vi "Finish.vi"   [LabVIEW 2014]
doc: "This VI is called just before exiting. It is expected to close I/O refnum, save collected data, etc."
uses:
  <vilib>/Rock Robotics/WPI/Joystick/WPI_JoystickGetSetRefNum.vi
  <vilib>/Rock Robotics/WPI/RobotDrive/WPI_RobotDriveGetSetRefNum.vi
types:
  T1 = typedef "WPI_JoystickDevRef.ctl" = cluster{"Device":T2}
  T2 = typedef "WPI_JoystickDeviceEnum.ctl" = enum16{"USB 0", "USB 1", "USB 2", "USB 3", "USB 4", "USB 5"}
  T3 = typedef "WPI_RobotDriveDevRef.ctl" = cluster{"DevStatus":errorcluster, "Motors[]":T4[], "Square Inputs":bool, "Max Output":dbl}
  T4 = typedef "WPI_MotorControlDeviceRef.ctl" = cluster{"DeviceStatus":errorcluster, "Type":T5, "PWM":cluster{"Controller":T6, "PWM Channel":T7, "DeadBand":T8}, "CAN":cluster{"Device Number":u8, "Control Mode":T9, "Semaphore":T10, "Max Vout":dbl, "TalonSRX Control Mode":T11}, "Invert":bool, "TransformRef":T12, "InvTransformRef":T12}
  T5 = typedef "WPI_MotorControlType.ctl" = enum16{"PWM", "CAN", "CANTalonSRX"}
  T6 = typedef "FPGA_TypedefDigitalModule.ctl" = enum16{"Controller 1"}
  T7 = typedef "FPGA_DIOPWMChannel.ctl" = enum8{"PWM 0", "PWM 1", "PWM 2", "PWM 3", "PWM 4", "PWM 5", "PWM 6", "PWM 7", "PWM 8", "PWM 9", "PWM MXP 0", "PWM MXP 1", "PWM MXP 2", "PWM MXP 3", "PWM MXP 4", "PWM MXP 5", "PWM MXP 6", "PWM MXP 7", "PWM MXP 8", "PWM MXP 9", "Invalid"}
  T8 = typedef "WPI_PWMDeadband.ctl" = cluster{"Name":string, "maxPositivePwm":i32, "minPositivePwm":i32, "centerPwm":i32, "maxNegativePwm":i32, "minNegativePwm":i32, "angularRange":u16}
  T9 = typedef "WPI_CANJaguar_ControlMode.ctl" = enum8{"Percent VBus", "Current", "Speed", "Position", "Voltage"}
  T10 = typedef "Semaphore RefNum" = refnum<k1>
  T11 = typedef "WPI_CANTalonSRX_APIControlMode.ctl" = enum8{"Percent VBus", "Speed", "Position", "Slave", "Unchanged / Invalid"}
  T12 = typedef "WPI_PWMTransform_ConPane.ctl" = refnum<vi>
  T13 = typedef "WPI_SolenoidDevRef.ctl" = cluster{"DevStatus":errorcluster, "Pneumatics Control Module":u8, "Forward Solenoid Channel":T14, "Reverse Solenoid Channel":T14}
  T14 = typedef "WPI_SolenoidChannel.ctl" = enum8{"Solenoid 0", "Solenoid 1", "Solenoid 2", "Solenoid 3", "Solenoid 4", "Solenoid 5", "Solenoid 6", "Solenoid 7", "Invalid"}
  T15 = typedef "WPI_SwitchDevRef.ctl" = cluster{"DevStatus":errorcluster, "DIO Channel":T16, "Controller":T6, "CntIndex":T17, "Normally Closed":bool}
  T16 = typedef "FPGA_DIOChannel.ctl" = enum8{"DIO 0", "DIO 1", "DIO 2", "DIO 3", "DIO 4", "DIO 5", "DIO 6", "DIO 7", "DIO 8", "DIO 9", "DIO MXP 0", "DIO MXP 1", "DIO MXP 2", "DIO MXP 3", "DIO MXP 4", "DIO MXP 5", "DIO MXP 6", "DIO MXP 7", "DIO MXP 8", "DIO MXP 9", "DIO MXP 10", "DIO MXP 11", "DIO MXP 12", "DIO MXP 13", "DIO MXP 14", "DIO MXP 15", "Invalid"}
  T17 = typedef "FPGA_CounterCtrSystemIndex.ctl" = enum8{"Ctr 0", "Ctr 1", "Ctr 2", "Ctr 3", "Ctr 4", "Ctr 5", "Ctr 6", "Ctr 7", "Invalid"}
  T18 = typedef "WPI_EncoderDevRef.ctl" = cluster{"DevStatus":errorcluster, "EncoderIndex":T19, "CounterIndex":T17, "DistancePerCount":dbl, "Decoding Type":T20}
  T19 = typedef "FPGA_EncoderIdx.ctl" = enum8{"Enc 0", "Enc 1", "Enc 2", "Enc 3", "Enc 4", "Enc 5", "Enc 6", "Enc 7", "Invalid"}
  T20 = typedef "WPI_EncoderType.ctl" = enum16{"1x", "2x", "4x"}
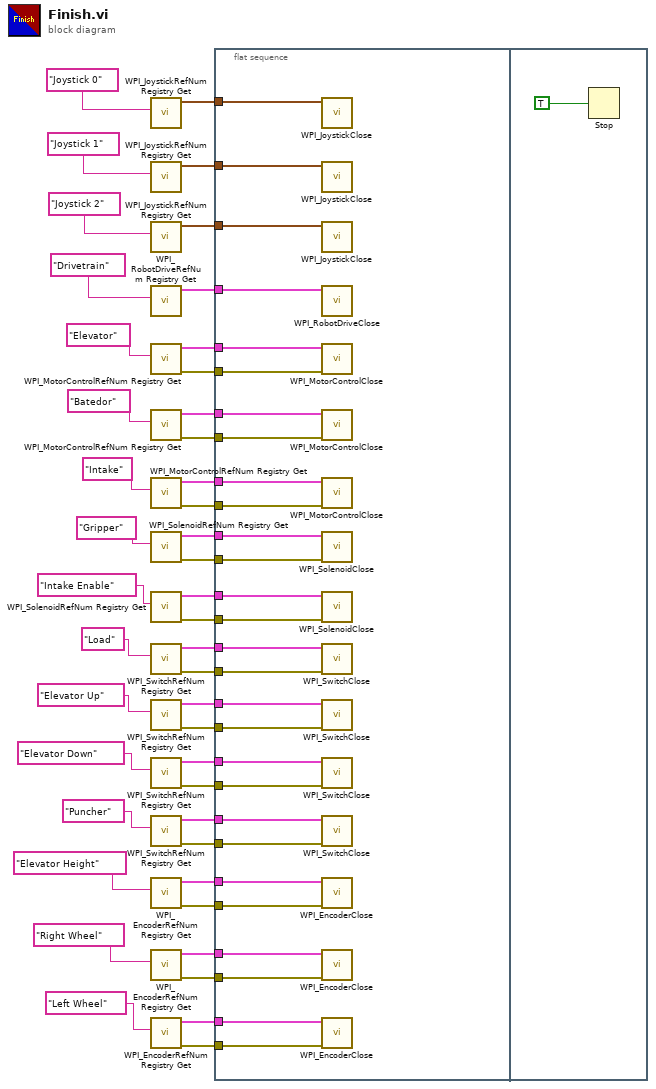
[diagram p0: block diagram]
diagram:
  n1 = call <vilib>:"WPI_JoystickRefNum Registry Get.vi"("refnum name"="Joystick 0") -> ("JoystickDevRef"=w41:T1)  [unwired: 1 in, 9 out]
  n2 = call <vilib>:"WPI_JoystickRefNum Registry Get.vi"("refnum name"="Joystick 1") -> ("JoystickDevRef"=w40:T1)  [unwired: 1 in, 9 out]
  n3 = call <vilib>:"WPI_JoystickRefNum Registry Get.vi"("refnum name"="Joystick 2") -> ("JoystickDevRef"=w37:T1)  [unwired: 1 in, 9 out]
  n4 = call <vilib>:"WPI_RobotDriveRefNum Registry Get.vi"("refnum name"="Drivetrain") -> ("RobotDriveDevRef"=w42:T3)  [unwired: 1 in, 9 out]
  n5 = call <vilib>:"WPI_MotorControlRefNum Registry Get.vi"("refnum name"="Elevator") -> ("error out"=w35:errorcluster, "MotorControlDevRef"=w36:T4)  [unwired: 9 in]
  n6 = call <vilib>:"WPI_MotorControlRefNum Registry Get.vi"("refnum name"="Batedor") -> ("error out"=w32:errorcluster, "MotorControlDevRef"=w31:T4)  [unwired: 9 in]
  n7 = call <vilib>:"WPI_MotorControlRefNum Registry Get.vi"("refnum name"="Intake") -> ("error out"=w29:errorcluster, "MotorControlDevRef"=w30:T4)  [unwired: 9 in]
  n8 = call <vilib>:"WPI_SolenoidRefNum Registry Get.vi"("refnum name"="Gripper") -> ("error out"=w27:errorcluster, "SolenoidDevRef"=w26:T13)  [unwired: 9 in]
  n9 = call <vilib>:"WPI_SolenoidRefNum Registry Get.vi"("refnum name"="Intake Enable") -> ("error out"=w23:errorcluster, "SolenoidDevRef"=w24:T13)  [unwired: 9 in]
  n10 = call <vilib>:"WPI_SwitchRefNum Registry Get.vi"("refnum name"="Load") -> ("error out"=w20:errorcluster, "SwitchDevRef"=w21:T15)  [unwired: 9 in]
  n11 = call <vilib>:"WPI_SwitchRefNum Registry Get.vi"("refnum name"="Elevator Up") -> ("error out"=w17:errorcluster, "SwitchDevRef"=w16:T15)  [unwired: 9 in]
  n12 = call <vilib>:"WPI_SwitchRefNum Registry Get.vi"("refnum name"="Elevator Down") -> ("error out"=w14:errorcluster, "SwitchDevRef"=w15:T15)  [unwired: 9 in]
  n13 = call <vilib>:"WPI_SwitchRefNum Registry Get.vi"("refnum name"="Puncher") -> ("error out"=w11:errorcluster, "SwitchDevRef"=w10:T15)  [unwired: 9 in]
  n14 = call <vilib>:"WPI_EncoderRefNum Registry Get.vi"("refnum name"="Elevator Height") -> ("error out"=w8:errorcluster, "EncoderDevRef"=w9:T18)  [unwired: 9 in]
  n15 = call <vilib>:"WPI_EncoderRefNum Registry Get.vi"("refnum name"="Right Wheel") -> ("error out"=w5:errorcluster, "EncoderDevRef"=w4:T18)  [unwired: 9 in]
  n16 = call <vilib>:"WPI_EncoderRefNum Registry Get.vi"("refnum name"="Left Wheel") -> ("error out"=w2:errorcluster, "EncoderDevRef"=w3:T18)  [unwired: 9 in]
  n17 = flat-sequence {
    tunnel: w42 -> [w72]
    tunnel: w41 -> [w71]
    tunnel: w40 -> [w70]
    tunnel: w37 -> [w69]
    tunnel: w36 -> [w68]
    tunnel: w35 -> [w67]
    tunnel: w31 -> [w65]
    tunnel: w32 -> [w66]
    tunnel: w30 -> [w64]
    tunnel: w29 -> [w63]
    tunnel: w27 -> [w62]
    tunnel: w26 -> [w61]
    tunnel: w23 -> [w59]
    tunnel: w24 -> [w60]
    tunnel: w21 -> [w58]
    tunnel: w20 -> [w57]
    tunnel: w16 -> [w55]
    tunnel: w17 -> [w56]
    tunnel: w15 -> [w54]
    tunnel: w14 -> [w53]
    tunnel: w10 -> [w51]
    tunnel: w11 -> [w52]
    tunnel: w9 -> [w50]
    tunnel: w8 -> [w49]
    tunnel: w4 -> [w47]
    tunnel: w5 -> [w48]
    tunnel: w3 -> [w46]
    tunnel: w2 -> [w45]
    frame #0 {
      n18 = call <vilib>:"WPI_JoystickClose.vi"("JoystickDevRef"=w71) -> ()  [unwired: 11 out]
      n19 = call <vilib>:"WPI_JoystickClose.vi"("JoystickDevRef"=w70) -> ()  [unwired: 11 out]
      n20 = call <vilib>:"WPI_JoystickClose.vi"("JoystickDevRef"=w69) -> ()  [unwired: 11 out]
      n21 = call <vilib>:"WPI_RobotDriveClose.vi"("RobotDriveDevRef"=w72) -> ()  [unwired: 1 in, 10 out]
      n22 = call <vilib>:"WPI_MotorControlClose.vi"("error in (no error)"=w67, "MotorControlDevRef"=w68) -> ()  [unwired: 9 in, 1 out]
      n23 = call <vilib>:"WPI_MotorControlClose.vi"("error in (no error)"=w66, "MotorControlDevRef"=w65) -> ()  [unwired: 9 in, 1 out]
      n24 = call <vilib>:"WPI_MotorControlClose.vi"("error in (no error)"=w63, "MotorControlDevRef"=w64) -> ()  [unwired: 9 in, 1 out]
      n25 = call <vilib>:"WPI_SolenoidClose.vi"("error in (no error)"=w62, "SolenoidDevRef"=w61) -> ()  [unwired: 9 in, 1 out]
      n26 = call <vilib>:"WPI_SolenoidClose.vi"("error in (no error)"=w59, "SolenoidDevRef"=w60) -> ()  [unwired: 9 in, 1 out]
      n27 = call <vilib>:"WPI_SwitchClose.vi"("error in (no error)"=w57, "SwitchDevRef"=w58) -> ()  [unwired: 9 in, 1 out]
      n28 = call <vilib>:"WPI_SwitchClose.vi"("error in (no error)"=w56, "SwitchDevRef"=w55) -> ()  [unwired: 9 in, 1 out]
      n29 = call <vilib>:"WPI_SwitchClose.vi"("error in (no error)"=w53, "SwitchDevRef"=w54) -> ()  [unwired: 9 in, 1 out]
      n30 = call <vilib>:"WPI_SwitchClose.vi"("error in (no error)"=w52, "SwitchDevRef"=w51) -> ()  [unwired: 9 in, 1 out]
      n31 = call <vilib>:"WPI_EncoderClose.vi"("error in (no error)"=w49, "EncoderDevRef"=w50) -> ()  [unwired: 9 in, 1 out]
      n32 = call <vilib>:"WPI_EncoderClose.vi"("error in (no error)"=w48, "EncoderDevRef"=w47) -> ()  [unwired: 9 in, 1 out]
      n33 = call <vilib>:"WPI_EncoderClose.vi"("error in (no error)"=w45, "EncoderDevRef"=w46) -> ()  [unwired: 9 in, 1 out]
    }
    frame #1 {
      n34 = Stop(stop? (T)=TRUE ("Quit")) -> ()
    }
  }
